vi "Read Scale.vi"(8 "error in (no error)":errorcluster, 11 "Knob.lvclass in":refnum<class "Knob.lvclass">) -> (0 "error out":errorcluster, 2 "Scale":refnum<vi>, 3 "Knob.lvclass out":refnum<class "Knob.lvclass">)   [LabVIEW 2015, in "Knob.lvclass"]
uses:
  Knob.lvclass
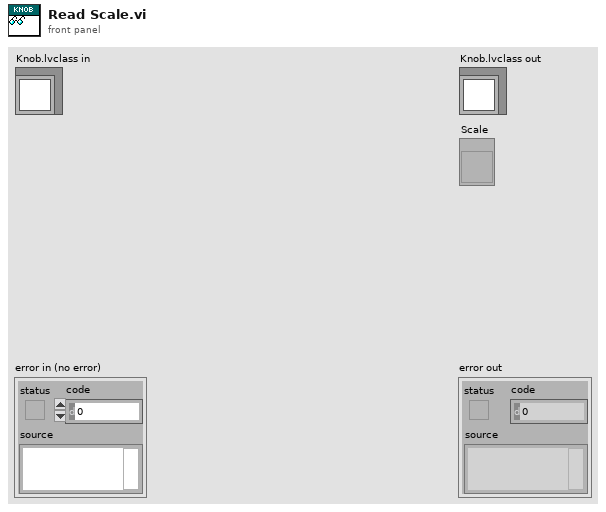
[diagram p1: front panel]
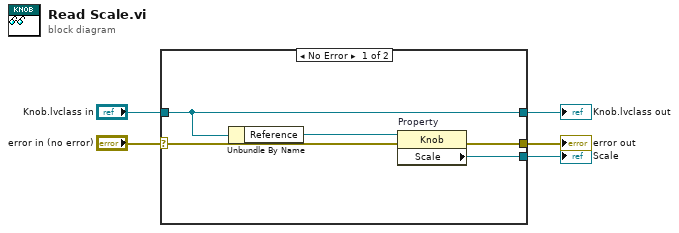
[diagram p0: block diagram]
diagram:
  n1 = case shown="No Error" "error in (no error)" {
    selector: "error in (no error)" -> [w6 w12]
    tunnel: [w9 w12] -> w4
    tunnel: [w8 w11] -> w2
    tunnel: "Knob.lvclass in" -> [w8 w11]
    tunnel: [w10 _] -> w1
    frame No Error {
      n2 = Unbundle By Name(w8) -> ("Reference"=w7:refnum<vi>)
      n3 = property on="Property" class="Knob"(reference=w7, error in=w6) -> (error out=w9:errorcluster, "Scale"=w10:refnum<vi>)  [unwired: 1 out]
    }
    frame Error {
    }
  }
  "error out" <- w4
  "Knob.lvclass out" <- w2
  "Scale" <- w1
